vi "Set_Speed.vi"(4 "Previous Tweaked demand":dbl format="%.2f", 5 "Channel Name (Calib Tweak)":string, 6 "Calib Tweak":dbl format="%.2f", 7 "Client Name":string, 8 "Channel Name (Volts/Amps)":string, 9 "Demanded Velocity":dbl format="%.2f", 10 "Channel Name (Velocity)":string) -> ()   [LabVIEW 2010]
uses:
  ADAM Client/Sub VIs/ADAM Controls/Update_scan_value.ctl
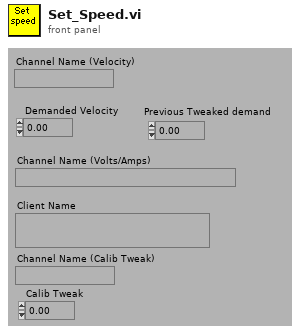
[diagram p1: front panel]
types:
  T1 = enum16{"Append to Global", "Read Global then Clear"}
  T2 = typedef "Update_scan_value.ctl" = cluster{"Channel Name":string, "New Value":dbl}
  T3 = typedef "Ch_description_ADAM.ctl" = cluster{"Ch Name":string, "Type":T4, "Function":T5, "Ch State":T6, "Calibration type":T7, "A":dbl, "B":dbl, "C":dbl, "D":dbl, "Comments":string, "Address":T8, "String":string, "Duty":u16}
  T4 = typedef "Module_type_ADAM.ctl" = enum16{"4011", "4012", "4013", "4014", "4016", "4017", "4018", "4021", "4050", "4052", "4053", "4060", "4080", "5000", "5017", "5018", "5024", "5051", "5056", "5060", "6060", "Tracker", "WEST", "GILL", "JEM", "VICI", "Vaisala", "DRUCK", "Run VI Named:", "IR2100", "PPT", "Comparator", "VIRTUAL", "Hold Value", "Read A", "Read Ch", "Coded", "Client Info", "Web Client", "X10", "Test"}
  T5 = typedef "Function_ADAM.ctl" = enum16{"Analogue Input", "Digital Input", "Event counter", "Event rate", "Analogue Output", "Digital Output", "Relay Output"}
  T6 = typedef "Channel_State.ctl" = enum16{"On", "Off", "Always On", "Always Off"}
  T7 = typedef "Calib_type_ADAM.ctl" = enum16{"Raw", "Bx + A", "Cx^2 + Bx + A", "Dx^3 + Cx^2 + Bx + A", "In Band", "Hi-Tec Q", "Hi-Tec M_dot", "Text"}
  T8 = typedef "Address.ctl" = cluster{"Main":i32, "Ch.":i32, "Sub":i32, "Port Name":string}
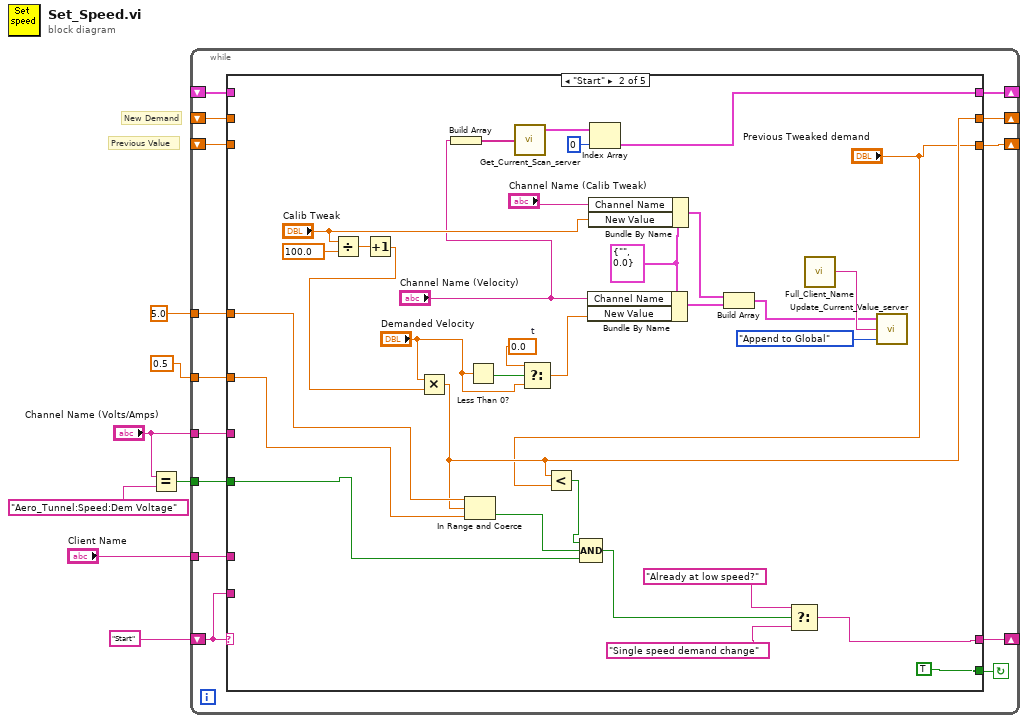
[diagram p0: block diagram]
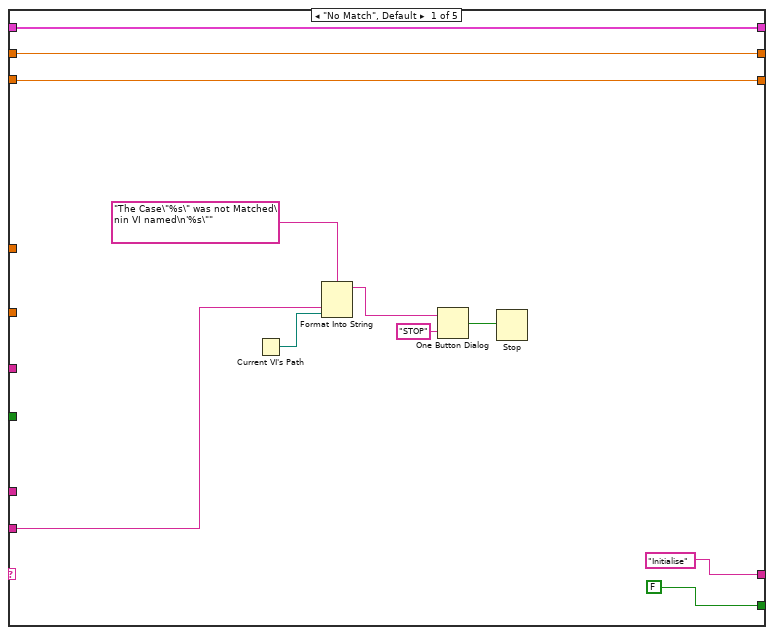
[diagram p2: hidden frame]
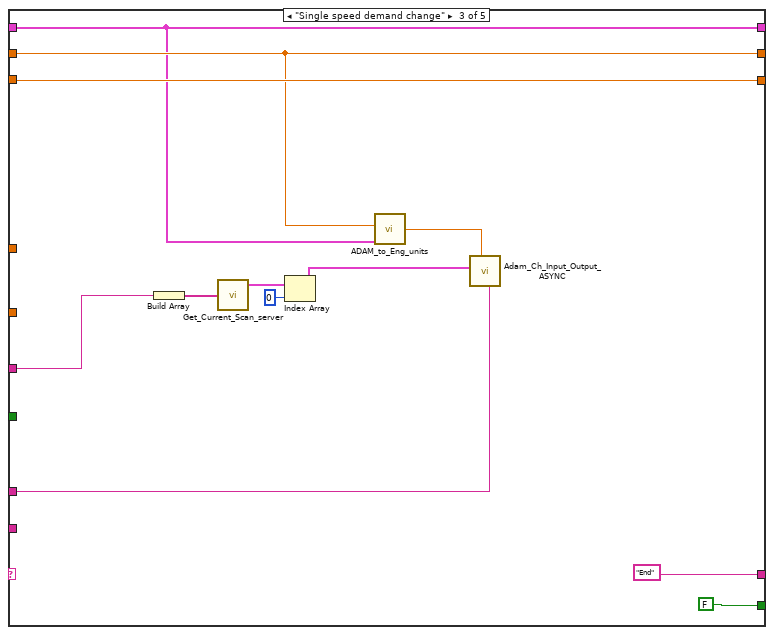
[diagram p3: hidden frame]
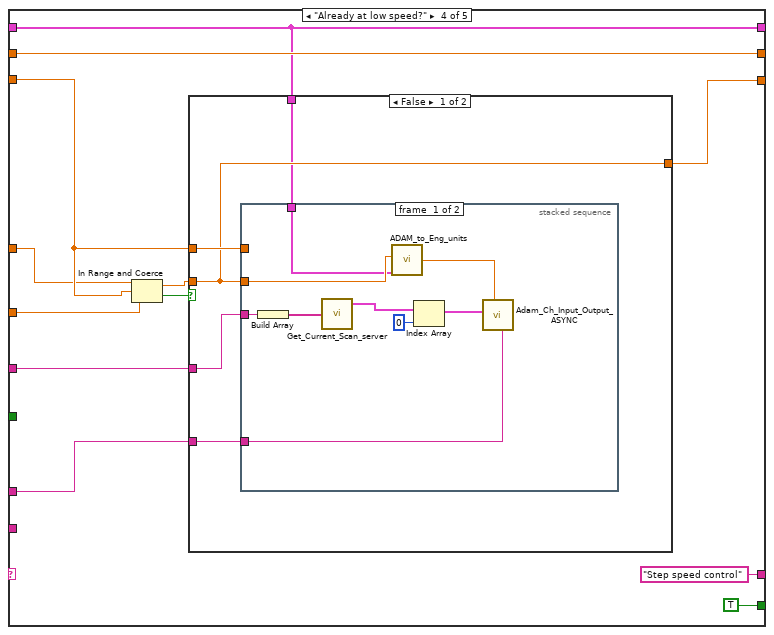
[diagram p4: hidden frame]
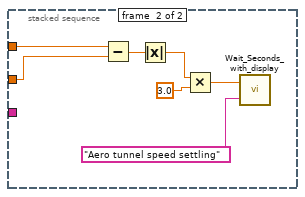
[diagram p5: hidden frame]
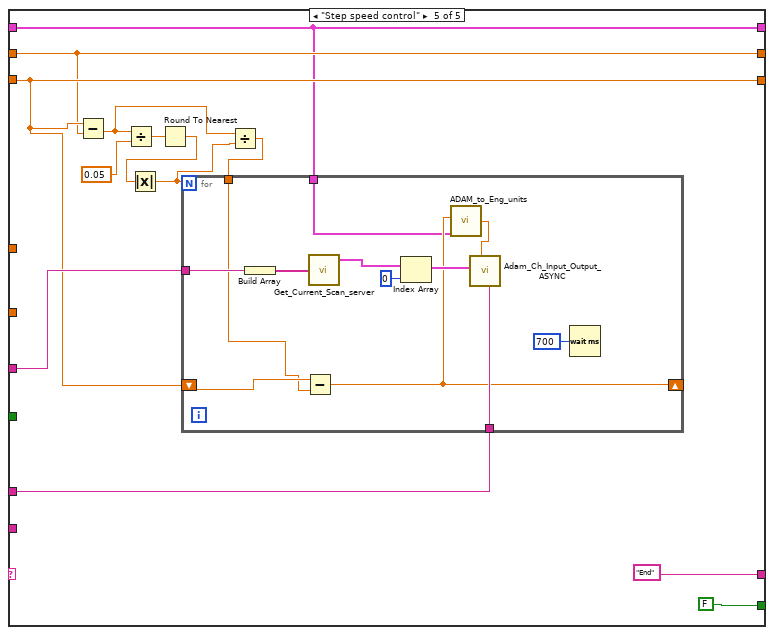
[diagram p7: hidden frame]
diagram:
  # "Previous Value"
  # "New Demand"
  n1 = Equal?(x="Channel Name (Volts/Amps)", y="Aero_Tunnel:Speed:Dem Voltage") -> (x = y?=w4:bool)
  n2 = while {
    shift-left: "Start" -> [w19]
    shift-right: [w20] -> _
    shift-right: [w16] -> _
    shift-left: _ -> [w17]
    tunnel: "Channel Name (Volts/Amps)" -> [w18]
    tunnel: w4 -> [w15]
    shift-right: [w14] -> _
    shift-left: _ -> [w13]
    tunnel: "Client Name" -> [w12]
    tunnel: 5.0 ("upper limit") -> [w11]
    tunnel: 0.5 ("lower limit") -> [w10]
    shift-right: [w9] -> _
    shift-left: _ -> [w8]
    stop <- w21 continue-if-true
    n3 = case shown="\"Start\"" w19 {
      tunnel: [FALSE TRUE FALSE TRUE FALSE] -> w21
      tunnel: ["Initialise" w47 "End" "Step speed control" "End"] -> w20
      tunnel: w19 -> [w27 _ _ _ _]
      tunnel: w18 -> [_ _ w71 w85 w121]
      tunnel: w17 -> [w24 _ w67 w88 w113]
      tunnel: [w24 w40 w67 w88 w113] -> w16
      tunnel: w15 -> [_ w45 _ _ _]
      tunnel: [w23 "Previous Tweaked demand" w70 w83 w114] -> w14
      tunnel: w13 -> [w23 _ w70 w84 w114]
      tunnel: w12 -> [_ _ w69 w82 w120]
      tunnel: w11 -> [_ w42 _ w79 _]
      tunnel: w10 -> [_ w41 _ w78 _]
      tunnel: [w22 w33 w65 w77 w111] -> w9
      tunnel: w8 -> [w22 _ w65 w77 w111]
      frame "No Match", Default {
        n4 = Current VI's Path() -> (path=w26:path)
        n5 = Format Into String(format string="The Case\"%s\" was not Matched\nin VI named\n'%s\"" ("Format String"), w27, w26) -> (resulting string=w30:string)  [unwired: 2 in, 1 out]
        n6 = One Button Dialog(message=w30, button name ("OK")="STOP") -> (true=w28:bool)
        n7 = Stop(stop? (T)=w28) -> ()
      }
      frame "Start" {
        w54 = T2 {"Channel Name"="", "New Value"=0.0} ("Update Scan Value Cluster")
        w60 = 0.0  # t
        n8 = Divide(x="Calib Tweak", y=100.0) -> (x/y=w59:dbl)
        n9 = Increment(x=w59) -> (x+1=w62:dbl)
        n10 = Multiply(x="Demanded Velocity", y=w62) -> (x*y=w40:dbl)
        n11 = Build Array("Channel Name (Velocity)") -> (w37:string[])
        n12 = In Range and Coerce(upper limit=w42, x=w40, lower limit=w41) -> (In Range?=w46:bool)  [unwired: 1 out]
        n13 = Less Than 0?(x="Demanded Velocity") -> (x < 0?=w52:bool)
        n14 = call "Get_Current_Scan_server.vi"("Desired Channels"=w37) -> ("Ch Description Array"=w34:T3[])  [unwired: 2 out]
        n15 = Select(t=w60, s=w52, f="Demanded Velocity") -> (s? t:f=w61:dbl)
        n16 = Less?(x=w40, y="Previous Tweaked demand") -> (x < y?=w38:bool)
        n17 = Compound Arithmetic op=AND(w38, w46, w45) -> (w44:bool)
        n18 = Bundle By Name(cluster=w54, "Channel Name"="Channel Name (Velocity)", "New Value"=w61) -> (w50:T2)
        n19 = Bundle By Name(cluster=w54, "Channel Name"="Channel Name (Calib Tweak)", "New Value"="Calib Tweak") -> (w56:T2)
        n20 = Index Array(array=w34, index=0) -> (element=w33:T3)
        n21 = Build Array(w56, w50) -> (w51:T2[])
        n22 = Select(t="Already at low speed?", s=w44, f="Single speed demand change") -> (s? t:f=w47:string)
        n23 = call "Full_Client_Name.vi"() -> ("Client Name"=w53:string)
        n24 = call "Update_Current_Value_server.vi"("Mode"=T1."Append to Global", "Client HD name"=w53, "Update array in"=w51) -> ()  [unwired: 1 out]
      }
      frame "Single speed demand change" {
        n25 = Build Array(w71) -> (w74:string[])
        n26 = call "Get_Current_Scan_server.vi"("Desired Channels"=w74) -> ("Ch Description Array"=w72:T3[])  [unwired: 2 out]
        n27 = Index Array(array=w72, index=0 ("Index")) -> (element=w68:T3)
        n28 = call "ADAM_to_Eng_units.vi"("Ch Description"=w65, "Raw"=w67) -> ("Calibrated units"=w66:dbl)  [unwired: 4 out]
        n29 = call "Adam_Ch_Input_Output_ASYNC.vi"("Client Name"=w69, "Value to Output"=w66, "Ch Discription"=w68) -> ()  [unwired: 4 in, 5 out]
      }
      frame "Already at low speed?" {
        n30 = In Range and Coerce(upper limit=w79, x=w84, lower limit=w78) -> (coerced(x)=w86:dbl, In Range?=w87:bool)
        n31 = case shown="False" w87 {
          tunnel: w86 -> [w91 _]
          tunnel: w85 -> [w93 _]
          tunnel: w84 -> [w92 w110]
          tunnel: [w91 w110] -> w83
          tunnel: w82 -> [w90 _]
          tunnel: w77 -> [w89 _]
          frame False {
            n32 = stacked-sequence {
              tunnel: w93 -> [w98 _]
              tunnel: w91 -> [w96 w108]
              tunnel: w92 -> [_ w109]
              tunnel: w90 -> [w97 _]
              tunnel: w89 -> [w95 _]
              frame #0 {
                n33 = Build Array(w98) -> (w101:string[])
                n34 = call "Get_Current_Scan_server.vi"("Desired Channels"=w101) -> ("Ch Description Array"=w99:T3[])  [unwired: 2 out]
                n35 = call "ADAM_to_Eng_units.vi"("Ch Description"=w95, "Raw"=w96) -> ("Calibrated units"=w94:dbl)  [unwired: 4 out]
                n36 = Index Array(array=w99, index=0 ("Index")) -> (element=w102:T3)
                n37 = call "Adam_Ch_Input_Output_ASYNC.vi"("Client Name"=w97, "Value to Output"=w94, "Ch Discription"=w102) -> ()  [unwired: 4 in, 5 out]
              }
              frame #1 {
                n38 = Subtract(x=w109, y=w108) -> (x-y=w107:dbl)
                n39 = Absolute Value(x=w107) -> (abs(x)=w106:dbl)
                n40 = Multiply(x=w106, y=3.0) -> (x*y=w104:dbl)
                n41 = call "Wait_Seconds_with_display.vi"("Message"="Aero tunnel speed settling", "Seconds to wait"=w104) -> ()  [unwired: 2 out]
              }
            }
          }
          frame True {
          }
        }
      }
      frame "Step speed control" {
        n42 = Subtract(x=w114, y=w113) -> (x-y=w117:dbl)
        n43 = Divide(x=w117, y=0.05) -> (x/y=w118:dbl)
        n44 = Round To Nearest(number=w118) -> (nearest integer value=w116:dbl)
        n45 = Absolute Value(x=w116) -> (abs(x)=w112:dbl)
        n46 = Divide(x=w117, y=w112) -> (x/y=w115:dbl)
        n47 = for {
          N: w112 -> [_]
          tunnel: w121 -> [w131]
          tunnel: w120 -> [w130]
          tunnel: w115 -> [w127]
          shift-right: [w126] -> _
          shift-left: w114 -> [w128]
          tunnel: w111 -> [w125]
          n48 = Build Array(w131) -> (w134:string[])
          n49 = Subtract(x=w128, y=w127) -> (x-y=w126:dbl)
          n50 = call "Get_Current_Scan_server.vi"("Desired Channels"=w134) -> ("Ch Description Array"=w132:T3[])  [unwired: 2 out]
          n51 = Index Array(array=w132, index=0 ("Index")) -> (element=w135:T3)
          n52 = call "ADAM_to_Eng_units.vi"("Ch Description"=w125, "Raw"=w126) -> ("Calibrated units"=w124:dbl)  [unwired: 4 out]
          n53 = call "Adam_Ch_Input_Output_ASYNC.vi"("Client Name"=w130, "Value to Output"=w124, "Ch Discription"=w135) -> ()  [unwired: 4 in, 5 out]
          n54 = Wait (ms)(milliseconds to wait=u32 700) -> ()  [unwired: 1 out]
        }
      }
    }
  }
